vi "CalcFZones.vi"(0 "F- zones":i16=7, 1 "# rf points per line":i32, 3 "Radii (m)":sgl[](array[numeric])=[0.0, 0.00132, 0.00142, 0.0019, 0.002, 0.00236, 0.00245, 0.00275, 0.00285, 0.0031], 4 "ROC (m)":dbl=0.012, 5 "Sampling Rate":sgl, 6 "delay (mm)":sgl, 7 "# Elements":i16=5, 8 "Dual mode":bool, 9 "c (m/s)":i32=1500, 10 "Round to ROC?":bool, 11 "File index number":i32, 12 "One Way Receive":bool) -> (13 "zone size mm":dbl, 14 "FZones (m)":dbl[](array[numeric]), 15 "ZoneStart":sgl[](array[numeric]), 17 "ZoneShift":sgl[](array[numeric]), 18 "ZoneLength":sgl[](array[numeric]), 19 "IndexVals":sgl[](array[numeric]))   [LabVIEW 2022 SP3]
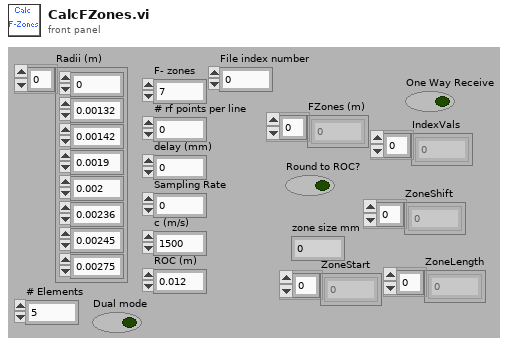
[diagram p1: front panel]
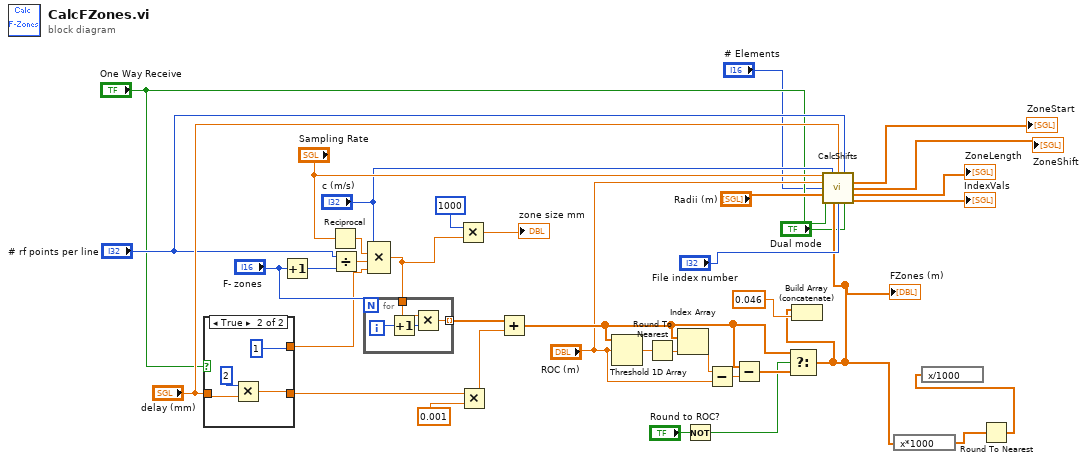
[diagram p0: block diagram]
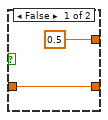
[diagram p2: hidden frame]
diagram:
  n1 = case shown="True" "One Way Receive" {
    tunnel: "delay (mm)" -> [w40 w42]
    tunnel: [w40 w43] -> w20
    tunnel: [0.5 1] -> w19
    frame False {
    }
    frame True {
      n2 = Multiply(x=2, y=w42) -> (x*y=w43:sgl)
    }
  }
  n3 = Increment(x="F- zones") -> (x+1=w28:i16)
  n4 = Reciprocal(x="Sampling Rate") -> (1/x=w33:sgl)
  n5 = Divide(x="# rf points per line", y=w28) -> (x/y=w29:dbl)
  n6 = Compound Arithmetic op=MULTIPLY("c (m/s)", w33, w29, w19) -> (w27:dbl)
  n7 = for {
    N: "F- zones" -> [_]
    tunnel: w27 -> [w48]
    tunnel: [w46] -> w36 mode=indexing
    i -> [w47]
    n8 = Increment(x=w47) -> (x+1=w45:i32)
    n9 = Multiply(x=w48, y=w45) -> (x*y=w46:dbl)
  }
  n10 = Multiply(x=1000, y=w27) -> (x*y=→"zone size mm":dbl)
  n11 = Multiply(x=w20, y=0.001) -> (x*y=w32:dbl)
  n12 = Add(x=w36, y=w32) -> (x+y=w23:dbl[])
  n13 = Threshold 1D Array(2:"ROC (m)", 3:w23) -> (0:w34:dbl)  [unwired: 1 out]
  n14 = Round To Nearest(number=w34) -> (nearest integer value=w37:dbl)
  n15 = Index Array(array=w23, index=w37) -> (element=w38:dbl)
  n16 = Not(x="Round to ROC?") -> (.not. x?=w21:bool)
  n17 = Subtract(x=w38, y="ROC (m)") -> (x-y=w35:dbl)
  n18 = Subtract(x=w23, y=w35) -> (x-y=w24:dbl[])
  n19 = Select(t=w23, s=w21, f=w24) -> (s? t:f=w3:dbl[])
  "FZones (m)" <- w3
  n20 = Build Array (concatenate)(w3, 0.046) -> ()  [unwired: 1 out]
  n21 = call "CalcShifts.vi"("Sampling Rate (Hz)"="Sampling Rate", "c (m/s)"="c (m/s)", "delay (mm)"="delay (mm)", "rf pts"="# rf points per line", "ROC (m)"="ROC (m)", "# Elements"="# Elements", "Radii (m)"="Radii (m)", "One Way Receive"="One Way Receive", "Focal lengths (m)"=w3, "File index number"="File index number", "Dual mode"="Dual mode") -> ("ZoneStart"=→"ZoneStart":sgl[], "ZoneShift"=→"ZoneShift":sgl[], "ZoneLength"=→"ZoneLength":sgl[], "IndexVals"=→"IndexVals":sgl[])  [unwired: 1 in]
  n22 = expression code="x*1000"(w3) -> (w6:dbl[])
  n23 = Round To Nearest(number=w6) -> (nearest integer value=w5:dbl[])
  n24 = expression code="x/1000"(w5) -> ()  [unwired: 1 out]
